vi "Read Charact Standard List.vi"(8 "error in (no error)":errorcluster, 11 "Path Group in":refnum<class "Path Group.lvclass">) -> (0 "error out":errorcluster, 2 "Charact Standard List":T1[](array[typedef]), 3 "Path Group out":refnum<class "Path Group.lvclass">)   [LabVIEW 2023, in "RFCalAndFixtureCharact.Common.lvlib" / "Path Group.lvclass"]
uses:
  Path Group.lvclass
  Fixture/Instruments/Cal Standard/Type Definitions/Standard Type.ctl
  Path Group.lvclass/Path Group.ctl
  Fixture/Instruments/RFFixtureCharact.Instruments.lvlib
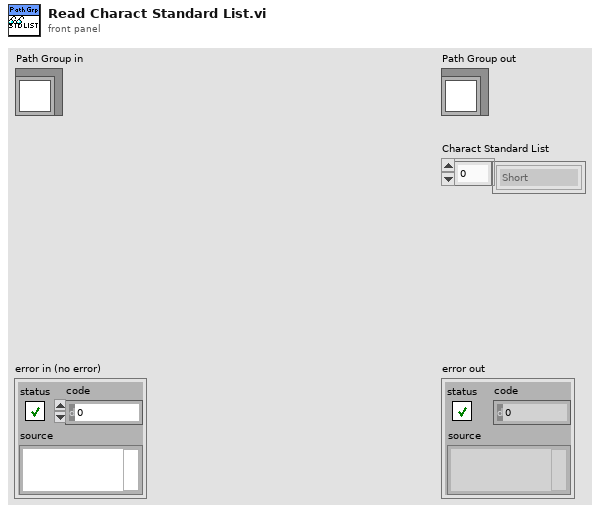
[diagram p1: front panel]
types:
  T1 = typedef "RFFixtureCharact.Instruments.lvlib/Standard Type.ctl" = enum16{"Short", "Open", "Load", "PowerMeter", "None"}
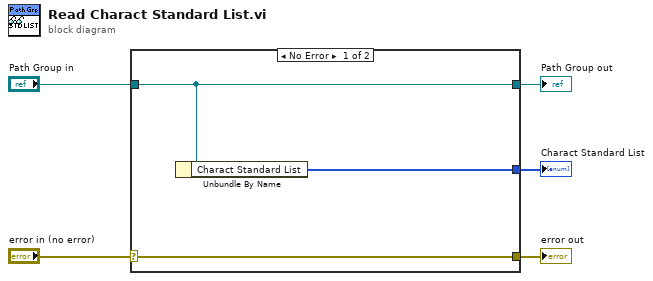
[diagram p0: block diagram]
diagram:
  n1 = case shown="No Error" "error in (no error)" {
    selector: "error in (no error)" -> [w8 w9]
    tunnel: [w8 w9] -> w4
    tunnel: [w7 w10] -> w2
    tunnel: "Path Group in" -> [w7 w10]
    tunnel: [w6 _] -> w1
    frame No Error {
      n2 = Unbundle By Name(w7) -> ("Charact Standard List"=w6:T1[])
    }
    frame Error {
    }
  }
  "error out" <- w4
  "Path Group out" <- w2
  "Charact Standard List" <- w1
